vi "TKPS252XG Reset24.vi"(2 "error in (no error)":errorcluster, 3 "VISA session":refnum<visa-resource-name>) -> (0 "error out":errorcluster, 1 "dup VISA session":refnum<visa-resource-name>)   [LabVIEW 2024]
doc: "This VI causes the instrument to reset. Consult the user's manual for the default parameter settings to which this command resets the instrument."
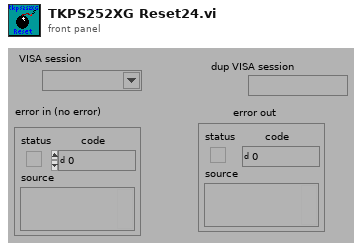
[diagram p1: front panel]
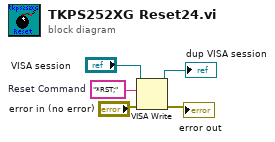
[diagram p0: block diagram]
diagram:
  w5 = "*RST;"  # Reset Command
  n1 = VISA Write(VISA resource name="VISA session", write buffer=w5, error in (no error)="error in (no error)") -> (VISA resource name out=→"dup VISA session":refnum<visa-resource-name>, error out=→"error out":errorcluster)  [unwired: 1 out]
